vi "add_installer_location-single.vi"(8 "error in (no error)":errorcluster, 11 "path":path) -> (0 "error out":errorcluster)   [LabVIEW 2015, in "lv-post-installer.lvlib"]
uses:
  lv-post-installer.lvlib
  private/_controls/fg_command.ctl
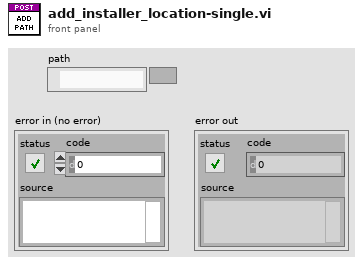
[diagram p1: front panel]
types:
  T1 = typedef "lv-post-installer.lvlib/fg_command.ctl" = enum16{"null", "initialize", "read", "write", "shutdown"}
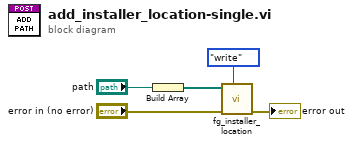
[diagram p0: block diagram]
diagram:
  n1 = Build Array("path") -> (w1:path[])
  n2 = call "fg_installer_location.vi"("fg_command"=fg_command."write", "error in (no error)"="error in (no error)", "path [] in"=w1) -> ("error out"=→"error out":errorcluster)  [unwired: 7 in, 1 out]
